vi "条件查找数组元素(2D DBL).vi"(8 "error in (no error)":errorcluster caption="错误输入（无错误）", 10 "条件数组":bool[][](array[boolean]), 11 "输入数组":dbl[][](array[numeric])) -> (0 "error out":errorcluster caption="错误输出", 2 "匹配元素索引":cluster{"行":i32, "列":i32}[](array[cluster]), 3 "符合条件元素":dbl[](array[numeric]) format="%.2f")   [LabVIEW 2011]
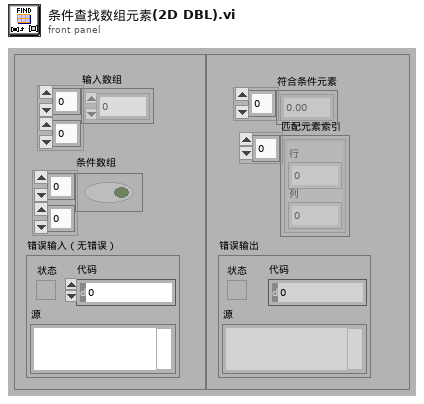
[diagram p1: front panel]
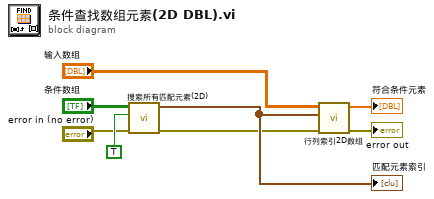
[diagram p0: block diagram]
diagram:
  n1 = call-poly "搜索所有匹配元素(2D).vi"("error in (no error)"="error in (no error)", "元素"=TRUE, "数组"="条件数组") -> ("error out"=w1:errorcluster, "匹配元素索引"=w3:cluster{"行":i32, "列":i32}[])  [unwired: 6 in, 1 out]
  "匹配元素索引" <- w3
  n2 = call-poly "行列索引2D数组.vi"("error in (no error)"=w1, "索引"=w3, "输入数组"="输入数组") -> ("error out"=→"error out":errorcluster, "元素"=→"符合条件元素":dbl[])  [unwired: 7 in]
